vi "Accumulate Waveform.vi"(8 "error in":errorcluster, 10 "Time to\n accumulate":dbl, 11 "Waveform":waveform(dbl)) -> (0 "error out":errorcluster, 3 "waveform out":waveform(dbl))   [LabVIEW 2024]
uses:
  <vilib>/Waveform/WDTOps.llb/WDT Append Waveforms DBL.vi
  <vilib>/Waveform/WDTOps.llb/WDT Get Waveform Subset DBL.vi
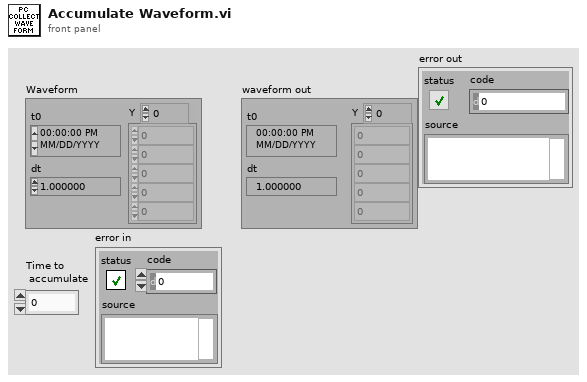
[diagram p1: front panel]
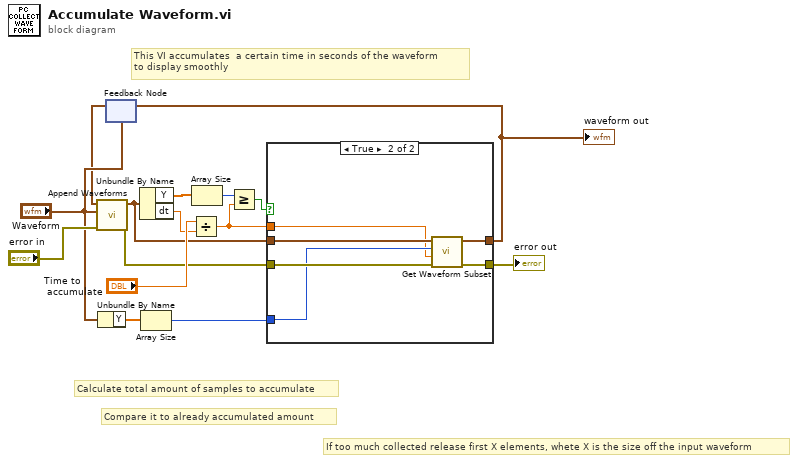
[diagram p0: block diagram]
diagram:
  # "If too much collected release first X elements, whete X is the size off the input waveform"
  # "Compare it to already accumulated amount"
  # "Calculate total amount of samples to accumulate"
  # "This VI accumulates  a certain time in seconds of the waveform \nto display smoothly"
  n1 = Unbundle By Name("Waveform") -> ("Y"=w14:dbl[])
  n2 = feedback #1("Waveform") -> (w4:waveform(dbl))
  n3 = call-poly <vilib>:"Append Waveforms.vi"("error in (no error)"="error in", "waveform B"="Waveform", "waveform A"=w4) -> ("error out"=w7:errorcluster, "waveform out"=w10:waveform(dbl))  [unwired: 7 in]
  n4 = Unbundle By Name(w10) -> ("Y"=w12:dbl[], "dt"=w9:dbl)
  n5 = Array Size(array=w14) -> (size(s)=w13:i32)
  n6 = Divide(x="Time to\n accumulate", y=w9) -> (x/y=w2:dbl)
  n7 = Array Size(array=w12) -> (size(s)=w3:i32)
  n8 = Greater Or Equal?(x=w3, y=w2) -> (x >= y?=w15:bool)
  n9 = case shown="True" w15 {
    tunnel: w10 -> [w17 w23]
    tunnel: [w17 w22] -> w1
    tunnel: w13 -> [_ w19]
    tunnel: w7 -> [w16 w21]
    tunnel: [w16 w20] -> w6
    tunnel: w2 -> [_ w18]
    frame False {
    }
    frame True {
      n10 = call-poly <vilib>:"Get Waveform Subset.vi"("error in (no error)"=w21, "duration"=w18, "start samples/time"=w19, "waveform in"=w23) -> ("error out"=w20:errorcluster, "waveform out"=w22:waveform(dbl))  [unwired: 2 in, 2 out]
    }
  }
  "waveform out" <- w1
  "error out" <- w6
  n11 = feedback-in #1(w1) -> ()
